vi "Close Network Engine.vi"(8 "error in (no error)":errorcluster, 10 "Parameters":T1 {"Config"."Industrial Settings"."Write Refs"."Data Reference" format="%.0x"; "Config"."Industrial Settings"."Read Refs"."Data Reference" format="%.0x"; "Config"."PID Settings"."Read Refs"."Data Reference" format="%.0x"; "Config"."PID Settings"."Write Refs"."Data Reference" format="%.0x"}, 11 "State Variables":T9) -> (0 "error out":errorcluster)   [LabVIEW 2019, in "Control Addon Engine.lvlib"]
uses:
  Control Addon Engine.lvlib
  Types/Network Engine State Variables.ctl
  <vilib>/NI/NIVS Inline Async API/_VS Inline Async API/Process/Process.lvclass
  <vilib>/NI/NI VeriStand Addon Network Comm/Engine/VeriStand Comm.lvclass
  Types/RT Configuration.ctl
  Addon Shared/Types/Gain Schedule.ctl
  Addon Shared/Types/Compiled Settings.ctl
  Addon Shared/Types/Compiled PID Settings.ctl
  <vilib>/NI VeriStand/Custom Device API/Block Data Reference.ctl
  <vilib>/NI VeriStand/Custom Device API/Data Reference.ctl
  Addon Shared/Types/Compiled Industrial Settings.ctl
  Addon Shared/Types/Compiled Industrial Parameters.ctl
  <vilib>/Utility/SystemLogging/Write to System Log.vi
  Addon Shared/Control Addon Shared.lvlib
  <vilib>/NI VeriStand/Custom Device API/Custom Device API.lvlib
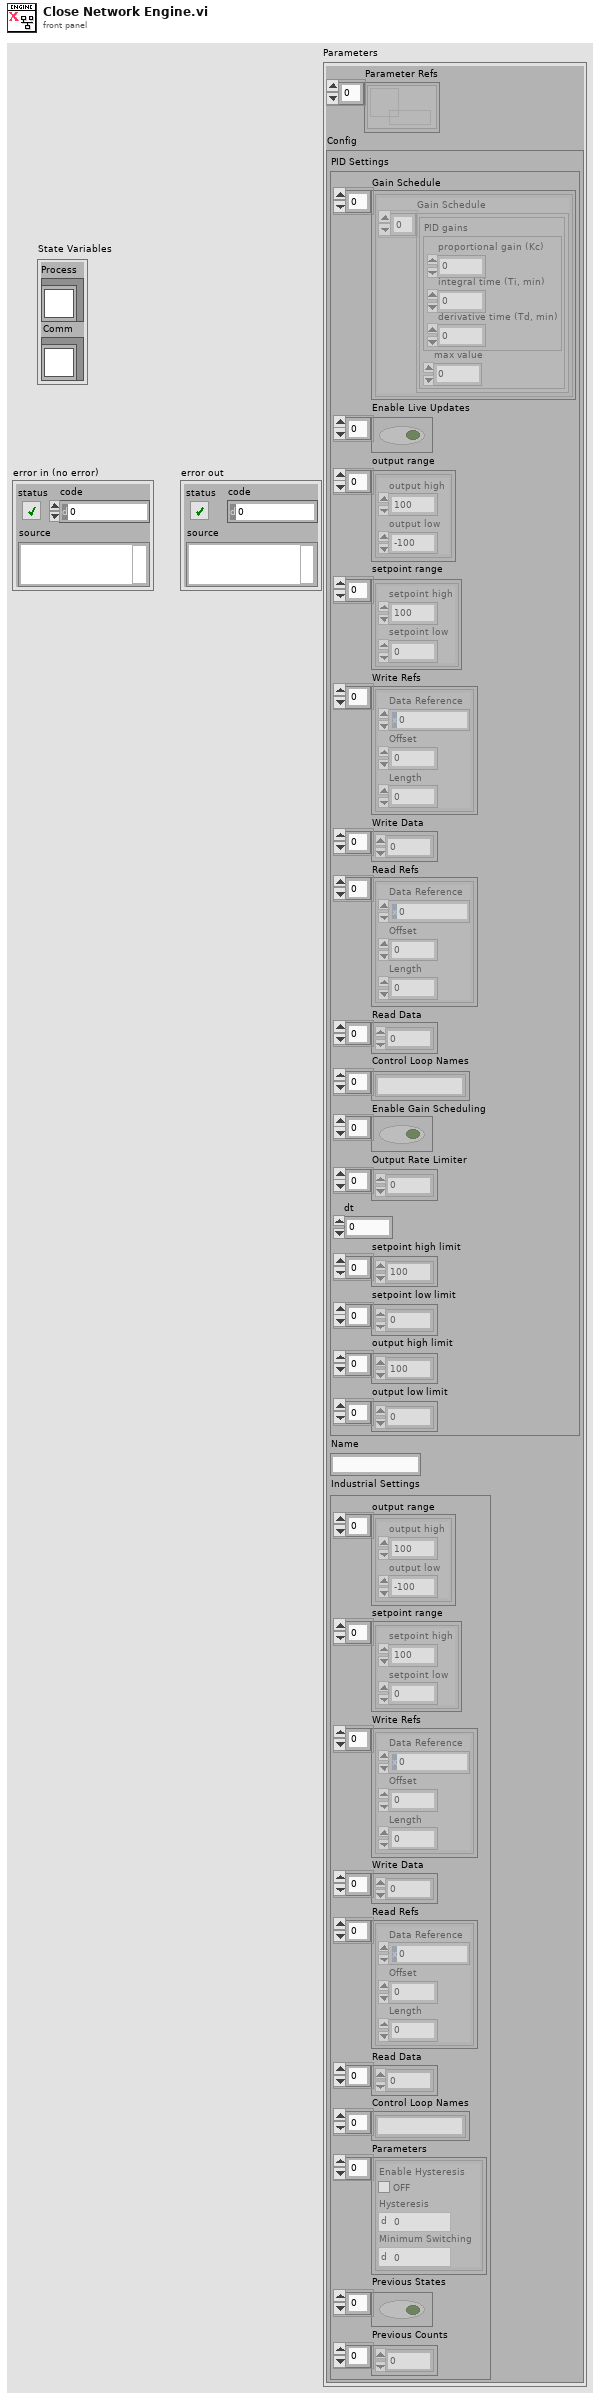
[diagram p1: front panel]
types:
  T1 = typedef "Control Addon Engine.lvlib/RT Configuration.ctl" = cluster{"Parameter Refs":refnum<data-value>[], "Config":T2}
  T2 = typedef "Control Addon Shared.lvlib/Compiled Settings.ctl" = cluster{"PID Settings":T3, "Name":string, "Industrial Settings":T7}
  T3 = typedef "Control Addon Shared.lvlib/Compiled PID Settings.ctl" = cluster{"Gain Schedule":T4[], "Enable Live Updates":bool[], "output range":cluster{"output high":dbl, "output low":dbl}[], "setpoint range":cluster{"setpoint high":dbl, "setpoint low":dbl}[], "Write Refs":T5[], "Write Data":dbl[], "Read Refs":T5[], "Read Data":dbl[], "Control Loop Names":string[], "Enable Gain Scheduling":bool[], "Output Rate Limiter":dbl[], "dt":dbl, "setpoint high limit":dbl[], "setpoint low limit":dbl[], "output high limit":dbl[], "output low limit":dbl[]}
  T4 = typedef "Control Addon Shared.lvlib/Gain Schedule.ctl" = cluster{"Gain Schedule":cluster{"PID gains":cluster{"proportional gain (Kc)":dbl, "integral time (Ti, min)":dbl, "derivative time (Td, min)":dbl}, "max value":dbl}[]}
  T5 = typedef "Custom Device API.lvlib/Block Data Reference.ctl" = cluster{"Data Reference":T6, "Offset":u64, "Length":u64}
  T6 = typedef "Custom Device API.lvlib/Data Reference.ctl" = i32
  T7 = typedef "Control Addon Shared.lvlib/Compiled Industrial Settings.ctl" = cluster{"output range":cluster{"output high":dbl, "output low":dbl}[], "setpoint range":cluster{"setpoint high":dbl, "setpoint low":dbl}[], "Write Refs":T5[], "Write Data":dbl[], "Read Refs":T5[], "Read Data":dbl[], "Control Loop Names":string[], "Parameters":T8[], "Previous States":bool[], "Previous Counts":u64[]}
  T8 = typedef "Control Addon Shared.lvlib/Compiled Industrial Parameters.ctl" = cluster{"Enable Hysteresis":bool, "Hysteresis":dbl, "Minimum Switching":u64}
  T9 = typedef "Control Addon Engine.lvlib/Network Engine State Variables.ctl" = cluster{"Process":refnum<class "Process.lvclass">, "Comm":refnum<class "VeriStand Comm.lvclass">}
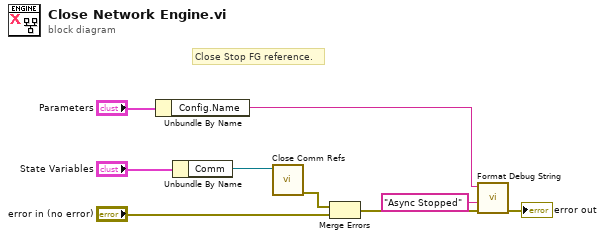
[diagram p0: block diagram]
diagram:
  # "Close Stop FG reference."
  n1 = Unbundle By Name("Parameters") -> ("Config.Name"=w1:string)
  n2 = Unbundle By Name("State Variables") -> ("Comm"=w6:refnum<class "VeriStand Comm.lvclass">)
  n3 = call <vilib>:"Close Comm Refs.vi"("Comm.lvclass"=w6) -> ("error out"=w8:errorcluster)  [unwired: 10 in]
  n4 = Merge Errors(w8, "error in (no error)") -> (w4:errorcluster)
  n5 = call "Format Debug String.vi"("error in (no error)"=w4, "State"="Async Stopped", "Name"=w1) -> ("error out"=→"error out":errorcluster)  [unwired: 8 in]
